vi "send move to stage GS.vi"(8 "error in (no error)":errorcluster, 10 "absolute position":dbl[unit], 11 "Autofocus in":refnum<class "Autofocus.lvclass">) -> (0 "error out":errorcluster, 3 "Autofocus out":refnum<class "Autofocus.lvclass">)   [LabVIEW 2012, in "Autofocus.lvclass"]
uses:
  Autofocus.lvclass
  <vilib>/Distrio/Murmex/GenericMessage/GenericMessage.lvclass
  Autofocus.lvclass/Autofocus.ctl
  <vilib>/Distrio/Murmex/Message/Message.lvclass
  <vilib>/Distrio/Murmex/Murmex/Murmex.lvclass
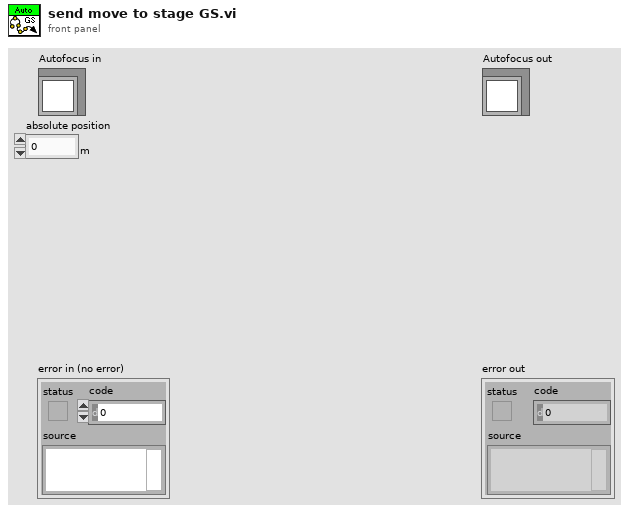
[diagram p1: front panel]
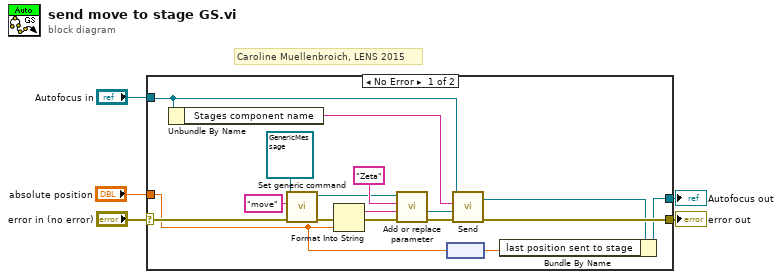
[diagram p0: block diagram]
diagram:
  # "Caroline Muellenbroich, LENS 2015"
  n1 = case shown="No Error" "error in (no error)" {
    selector: "error in (no error)" -> [w11 w24]
    tunnel: [w10 w24] -> w4
    tunnel: [w8 w23] -> w2
    tunnel: "Autofocus in" -> [w12 w23]
    tunnel: "absolute position" -> [w6 _]
    frame No Error {
      n2 = Unbundle By Name(w12) -> ("Stages component name"=w14:string)
      n3 = call <vilib>:"Set generic command.vi"("error in (no error)"=w11, "generic command"="move" ("command string"), "GenericMessage in"=refnum<class "GenericMessage.lvclass"> refnum ("Murmex.lvlib:GenericMessage")) -> ("error out"=w15:errorcluster, "GenericMessage out"=w13:refnum<class "GenericMessage.lvclass">)  [unwired: 7 in]
      n4 = Format Into String(error in=w15, w6) -> (resulting string=w19:string, error out=w18:errorcluster)  [unwired: 2 in]
      n5 = call <vilib>:"Add or replace parameter.vi"("error in (no error)"=w18, "value"=w19, "name"="Zeta", "Message in"=w13) -> ("error out"=w21:errorcluster, "Message out"=w22:refnum<class "GenericMessage.lvclass">)  [unwired: 6 in]
      n6 = node(w6) -> (w7:dbl)
      n7 = call <vilib>:"Send.vi"("error in (no error)"=w21, "Message"=w22, "recipient"=w14, "Murmex in"=w12) -> ("error out"=w10:errorcluster, "Murmex out"=w9:refnum<class "Autofocus.lvclass">)  [unwired: 6 in]
      n8 = Bundle By Name(cluster=w9, "last position sent to stage"=w7) -> (w8:refnum<class "Autofocus.lvclass">)
    }
    frame Error {
    }
  }
  "error out" <- w4
  "Autofocus out" <- w2
